vi "demo.vi"() -> ()   [LabVIEW 2021]
uses:
  bfa3c46e-401b-3fef-3c69-c7d7ae93e03f.vi
  52da8b2e-b3f7-3fe9-ec11-5ffec2ece33f.vi
  3f00d7fc-b427-3fef-b462-8341edb6e83f.vi
  b9595c78-9250-3fda-dc67-64190d2ce13f.vi
  81bbc9f6-d05f-3feb-bc58-e5c44a84e43f.vi
  fc065110-cdb9-3fd5-189f-eae20fa3d43f.vi
  90bbcc10-7294-3fcf-d098-d044dc92d63f.vi
  85ac1abc-bf5a-3fee-8080-d99c488dc33f.vi
  7bf0db12-82e5-3fe1-8006-8ac0b96fc63f.vi
  344c3781-5a31-3fdb-64f9-2935f1fdd13f.vi
  DoublyLinkedList/DoublyLinkedList.lvclass
  Iterator/Iterator.lvclass
panel:
  out "numbers":dbl[](array[numeric])
  out "strings":string[](array[string])
  out "error out":errorcluster
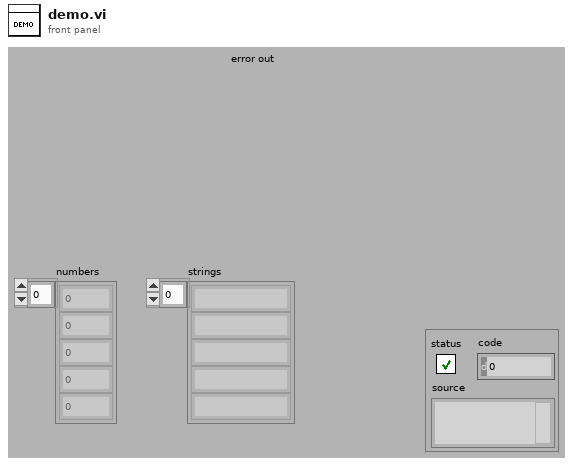
[diagram p1: front panel]
types:
  T1 = cluster{"DoublyLinkedList.lvclass":refnum<class "DoublyLinkedList.lvclass">, "element data type":dbl}
  T2 = cluster{"DoublyLinkedList.lvclass":refnum<class "DoublyLinkedList.lvclass">, "element data type":string}
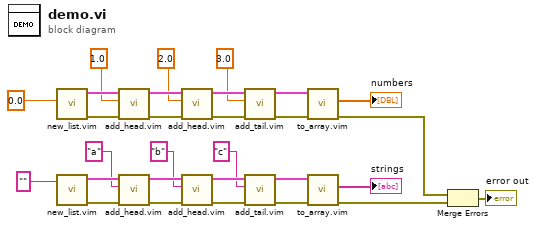
[diagram p0: block diagram]
diagram:
  n1 = call "new_list.vim"("element data type"=0.0 ("data")) -> ("error out"=w24:errorcluster, "new list"=w28:T1)  [unwired: 9 in]
  n2 = call "new_list.vim"("element data type"="") -> ("error out"=w11:errorcluster, "new list"=w15:T2)  [unwired: 9 in]
  n3 = call "add_head.vim"("error in (no error)"=w24, "element data type"=1.0 ("data"), "list in"=w28) -> ("error out"=w22:errorcluster, "list out"=w27:T1)  [unwired: 7 in]
  n4 = call "add_head.vim"("error in (no error)"=w11, "element data type"="a", "list in"=w15) -> ("error out"=w10:errorcluster, "list out"=w13:T2)  [unwired: 7 in]
  n5 = call "add_head.vim"("error in (no error)"=w22, "element data type"=2.0 ("data"), "list in"=w27) -> ("error out"=w19:errorcluster, "list out"=w26:T1)  [unwired: 7 in]
  n6 = call "add_head.vim"("error in (no error)"=w10, "element data type"="b", "list in"=w13) -> ("error out"=w7:errorcluster, "list out"=w9:T2)  [unwired: 7 in]
  n7 = call "add_tail.vim"("error in (no error)"=w19, "element data type"=3.0 ("data"), "list in"=w26) -> ("error out"=w18:errorcluster, "list out"=w25:T1)  [unwired: 7 in]
  n8 = call "add_tail.vim"("error in (no error)"=w7, "element data type"="c", "list in"=w9) -> ("error out"=w17:errorcluster, "list out"=w6:T2)  [unwired: 7 in]
  n9 = call "to_array.vim"("error in (no error)"=w18, "list in"=w25) -> ("error out"=w3:errorcluster, "data"=→"numbers":dbl[])  [unwired: 7 in, 1 out]
  n10 = call "to_array.vim"("error in (no error)"=w17, "list in"=w6) -> ("error out"=w2:errorcluster, "data"=→"strings":string[])  [unwired: 7 in, 1 out]
  n11 = Merge Errors(w3, w2) -> (→"error out":errorcluster)
